vi "ELVIS III v1.0 Unreserve Channel List Core.vi"(7 "Allow multiple opens?":bool, 8 "error in (no error)":errorcluster, 10 "Channel Reservation List":T1, 11 "Owner":string) -> (0 "error out":errorcluster)   [LabVIEW 2021]
uses:
  <vilib>/myRIO/Common/Instrument Driver Framework/ELVIS III v1.0/Resource Manager/typedefs/ELVIS III v1.0 Channel Reservation List.ctl
  <vilib>/myRIO/Common/Instrument Driver Framework/ELVIS III v1.0/Resource Manager/typedefs/ELVIS III v1.0 Channel Reservation Info.ctl
  <vilib>/myRIO/Common/Instrument Driver Framework/ELVIS III v1.0/Resource Manager/typedefs/ELVIS III v1.0 Connector List.ctl
  <vilib>/myRIO/Common/Instrument Driver Framework/ELVIS III v1.0/Resource Manager/vis/ELVIS III v1.0 Build Mutex Name.vi
  <vilib>/myRIO/Common/Instrument Driver Framework/Utilities/vis/Configuration Manager.vi
  <vilib>/myRIO/Common/Instrument Driver Framework/Utilities/vis/IO Manager.vi
  <vilib>/Utility/error.llb/Error Cluster From Error Code.vi
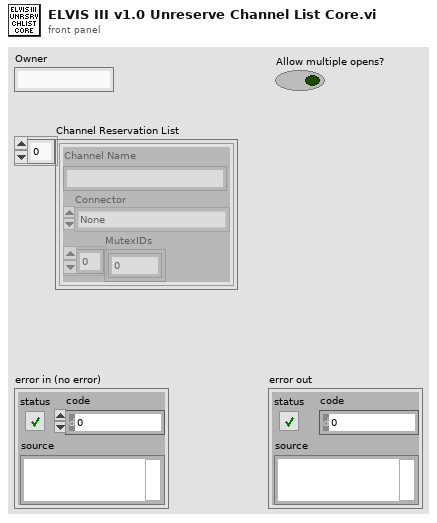
[diagram p1: front panel]
types:
  T1 = typedef "ELVIS III v1.0 Channel Reservation List.ctl" = T2[]
  T2 = typedef "ELVIS III v1.0 Channel Reservation Info.ctl" = cluster{"Channel Name":string, "Connector":T3, "MutexIDs":u32[]}
  T3 = typedef "ELVIS III v1.0 Connector List.ctl" = enum32{"None", "ConnectorA", "ConnectorB"}
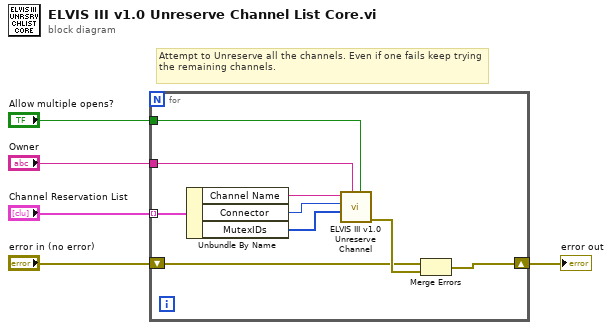
[diagram p0: block diagram]
diagram:
  # "Attempt to Unreserve all the channels. Even if one fails keep trying the remaining channels."
  n1 = for {
    tunnel: "Owner" -> [w12]
    tunnel: "Allow multiple opens?" -> [w13]
    tunnel: "Channel Reservation List" -> [w14] mode=indexing
    shift-right: [w6] -> w5
    shift-left: "error in (no error)" -> [w7]
    n2 = Unbundle By Name(w14) -> ("Channel Name"=w11:string, "Connector"=w10:T3, "MutexIDs"=w9:u32[])
    n3 = call <vilib>:"ELVIS III v1.0 Unreserve Channel.vi"("Allow multiple opens?"=w13, "Owner"=w12, "Mutex IDS"=w9, "Connector"=w10, "Channel Name"=w11) -> ("error out"=w8:errorcluster)  [unwired: 6 in]
    n4 = Merge Errors(w7, w8) -> (w6:errorcluster)
  }
  "error out" <- w5
